vi "xps_panel_update_current_position.vi"(8 "error in (no error)":errorcluster, 11 "newport_xps_panel in":refnum<class "newport_xps_panel.lvclass">) -> (0 "error out":errorcluster, 3 "newport_xps_panel out":refnum<class "newport_xps_panel.lvclass">)   [LabVIEW 2015, in "newport_xps_panel.lvclass"]
uses:
  newport_xps_panel.lvclass
  newport_xps/newport_xps.lvclass
  newport_xps_panel.lvclass/newport_xps_panel.ctl
  UI/panel_class/panel.lvclass
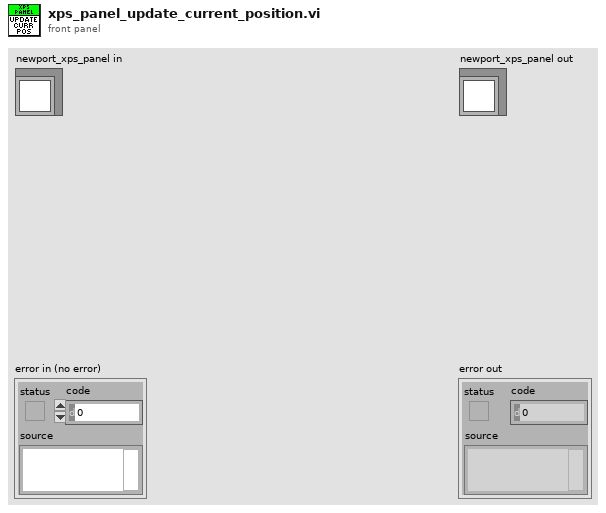
[diagram p1: front panel]
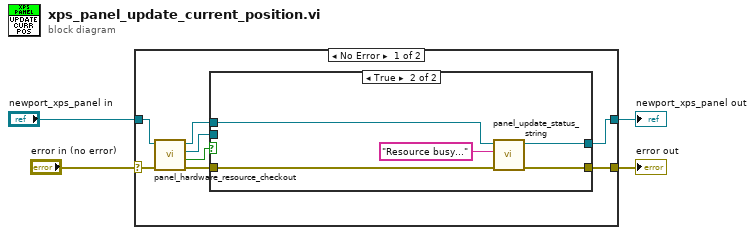
[diagram p0: block diagram]
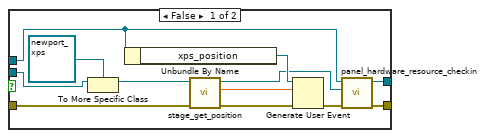
[diagram p2: hidden frame]
diagram:
  n1 = case shown="No Error" "error in (no error)" {
    selector: "error in (no error)" -> [w11 w31]
    tunnel: [w7 w31] -> w3
    tunnel: [w5 w30] -> w1
    tunnel: "newport_xps_panel in" -> [w12 w30]
    frame No Error {
      n2 = call "panel_hardware_resource_checkout.vi"("error in (no error)"=w11, "panel in"=w12) -> ("error out"=w10:errorcluster, "timed out?"=w6:bool, "hardware.lvclass"=w9:refnum<class "hardware.lvclass">, "panel out"=w8:refnum<class "newport_xps_panel.lvclass">)  [unwired: 6 in]
      n3 = case shown="True" w6 {
        tunnel: w10 -> [w24 w28]
        tunnel: w9 -> [w22 _]
        tunnel: w8 -> [w21 w27]
        tunnel: [w20 w26] -> w7
        tunnel: [w19 w25] -> w5
        frame False {
          n4 = To More Specific Class(target class=refnum<class "newport_xps.lvclass"> refnum ("newport_xps.lvclass"), reference=w22) -> (specific class reference=w18:refnum<class "newport_xps.lvclass">)  [unwired: 1 in, 1 out]
          n5 = Unbundle By Name(w21) -> ("xps_position"=w15:refnum<user-event>)
          n6 = call-dynamic "stage_get_position.vi"("error in (no error)"=w24, "newport_xps in"=w18) -> ("error out"=w17:errorcluster, "Position"=w14:dbl, "newport_xps out"=w13:refnum<class "newport_xps.lvclass">)  [unwired: 7 in]
          n7 = Generate User Event(user event=w15, event data cluster=w14, error in=w17) -> (error out=w16:errorcluster)  [unwired: 1 in, 1 out]
          n8 = call "panel_hardware_resource_checkin.vi"("error in (no error)"=w16, "hardware.lvclass"=w13, "panel in"=w21) -> ("error out"=w20:errorcluster, "panel out"=w19:refnum<class "newport_xps_panel.lvclass">)  [unwired: 7 in]
        }
        frame True {
          n9 = call-dynamic "panel_update_status_string.vi"("error in (no error)"=w28, "String"="Resource busy...", "newport_xps_panel in"=w27) -> ("error out"=w26:errorcluster, "newport_xps_panel out"=w25:refnum<class "newport_xps_panel.lvclass">)  [unwired: 7 in]
        }
      }
    }
    frame Error {
    }
  }
  "error out" <- w3
  "newport_xps_panel out" <- w1
